vi "Convert Excel Cell To Hour_Min  String.vi"(8 "error in (no error)":errorcluster, 10 "Hour:Min(\"\")":string, 11 "ExceelDate in":refnum<class "ExceelDate.lvclass">) -> (0 "error out":errorcluster, 2 "Hour:Min(\"\")":string, 3 "ExceelDate out":refnum<class "ExceelDate.lvclass">)   [LabVIEW 2015, in "ExceelDate.lvclass"]
uses:
  ExceelDate.lvclass
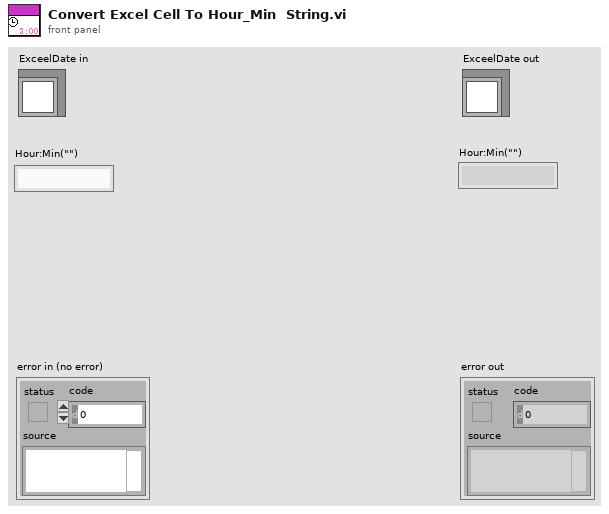
[diagram p1: front panel]
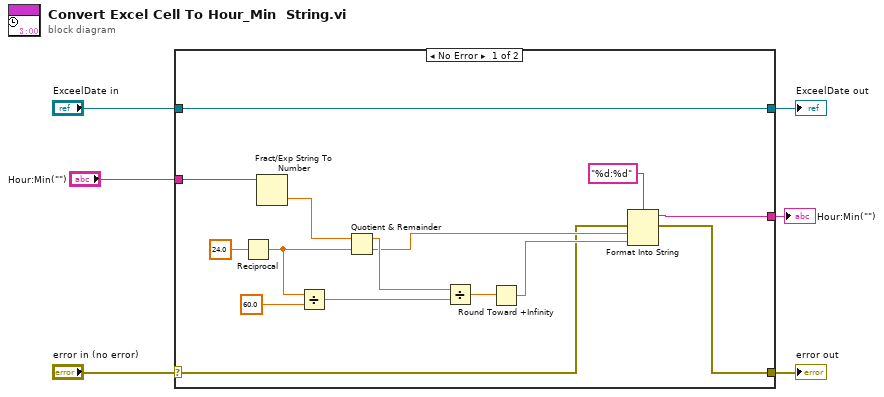
[diagram p0: block diagram]
diagram:
  n1 = case shown="No Error" "error in (no error)" {
    selector: "error in (no error)" -> [w8 w23]
    tunnel: [w7 w23] -> w5
    tunnel: [w21 w22] -> w3
    tunnel: "ExceelDate in" -> [w21 w22]
    tunnel: "Hour:Min(\"\")" -> [w20 _]
    tunnel: [w9 _] -> w1
    frame No Error {
      n2 = Reciprocal(x=24.0) -> (1/x=w17:dbl)
      n3 = Fract/Exp String To Number(string=w20) -> (number=w18:dbl)  [unwired: 3 in, 1 out]
      n4 = Divide(x=w17, y=60.0) -> (x/y=w15:dbl)
      n5 = Quotient & Remainder(x=w18, y=w17) -> (x-y*floor(x/y)=w13:dbl, floor(x/y)=w11:dbl)
      n6 = Divide(x=w13, y=w15) -> (x/y=w14:dbl)
      n7 = Round Toward +Infinity(x=w14) -> (ceil(x): smallest int >= x=w10:dbl)
      n8 = Format Into String(format string="%d:%d", error in=w8, w11, w10) -> (resulting string=w9:string, error out=w7:errorcluster)  [unwired: 1 in]
    }
    frame Error {
    }
  }
  "error out" <- w5
  "ExceelDate out" <- w3
  "Hour:Min(\"\")" <- w1
